vi "仁科设定参数对话框.vi"() -> ()   [LabVIEW 2016, in "环境动力监测库.lvlib" / "空调库.lvlib"]
panel:
  in  "帮助按钮":bool
  in  "时间 16":cluster{"小时":u16, "分钟":u16} {"分钟" format="%.0f分"; "小时" format="%.0f点"}
  in  "时间 15":cluster{"小时":u16, "分钟":u16} {"分钟" format="%.0f分"; "小时" format="%.0f点"}
  in  "时间 14":cluster{"小时":u16, "分钟":u16} {"分钟" format="%.0f分"; "小时" format="%.0f点"}
  in  "时间 13":cluster{"小时":u16, "分钟":u16} {"分钟" format="%.0f分"; "小时" format="%.0f点"}
  in  "时间 12":cluster{"小时":u16, "分钟":u16} {"分钟" format="%.0f分"; "小时" format="%.0f点"}
  in  "时间 11":cluster{"小时":u16, "分钟":u16} {"分钟" format="%.0f分"; "小时" format="%.0f点"}
  in  "时间 10":cluster{"小时":u16, "分钟":u16} {"分钟" format="%.0f分"; "小时" format="%.0f点"}
  in  "时间 9":cluster{"小时":u16, "分钟":u16} {"分钟" format="%.0f分"; "小时" format="%.0f点"}
  in  "时间 8":cluster{"小时":u16, "分钟":u16} {"分钟" format="%.0f分"; "小时" format="%.0f点"}
  in  "时间 7":cluster{"小时":u16, "分钟":u16} {"分钟" format="%.0f分"; "小时" format="%.0f点"}
  in  "时间 6":cluster{"小时":u16, "分钟":u16} {"分钟" format="%.0f分"; "小时" format="%.0f点"}
  in  "时间 5":cluster{"小时":u16, "分钟":u16} {"分钟" format="%.0f分"; "小时" format="%.0f点"}
  in  "时间 4":cluster{"小时":u16, "分钟":u16} {"分钟" format="%.0f分"; "小时" format="%.0f点"}
  in  "时间 3":cluster{"小时":u16, "分钟":u16} {"分钟" format="%.0f分"; "小时" format="%.0f点"}
  in  "时间 2":cluster{"小时":u16, "分钟":u16} {"分钟" format="%.0f分"; "小时" format="%.0f点"}
  in  "时间":cluster{"小时":u16, "分钟":u16} {"分钟" format="%.0f分"; "小时" format="%.0f点"}
  in  "通道2空调故障报警":bool
  in  "通道1空调故障报警":bool
  in  "低温报警":bool
  in  "超温报警":bool
  in  "空调电流门槛:":dbl
  in  "湿度偏差:":dbl
  in  "温度偏差:":dbl
  in  "自控温度回差:":dbl
  in  "自控温度下限:":dbl
  in  "温度报警下限:":dbl
  in  "自控温度上限:":dbl
  in  "温度报警上限:":dbl
  in  "切换时间(分钟):":dbl
  in  "双机切换":bool
  in  "控制模式:":enum16{"远程", "自动"}(ring)
  in  "来电自启":bool
  in  "写入控制参数":bool
  in  "读取运行参数":bool
  # "设定参数选择"
  # "通道运行时间段"
  # "时间段1"
  # "时间段2"
  # "时间段3"
  # "时间段4"
  # "通道1开始:"
  # "通道1结束:"
  # "通道2开始:"
  # "通道2结束:"
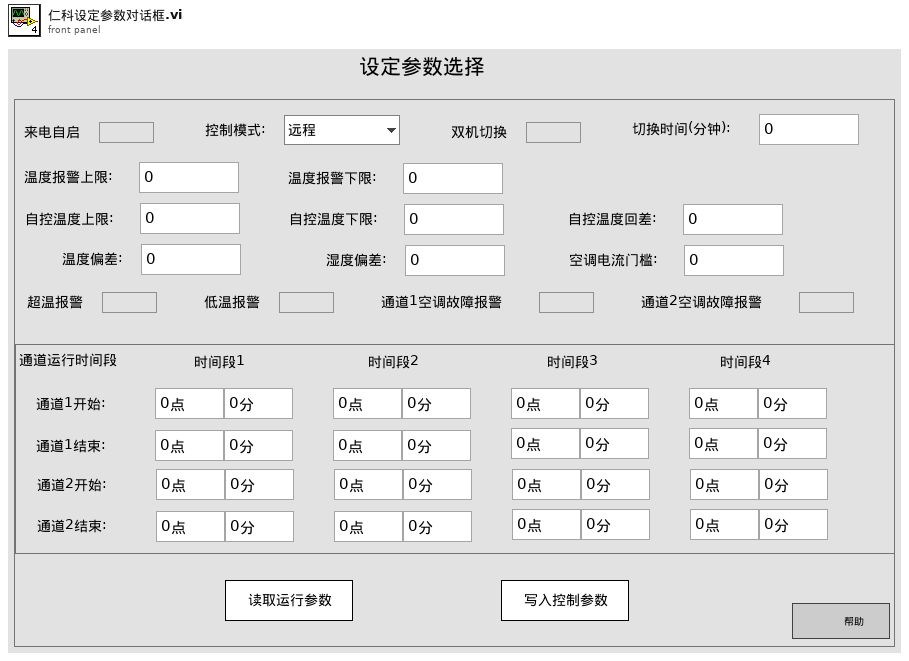
[diagram p1: front panel]
types:
  T1 = cluster{"来电自启":bool, "时间":cluster{"小时":u16, "分钟":u16}, "时间 2":cluster{"小时":u16, "分钟":u16}, "时间 3":cluster{"小时":u16, "分钟":u16}, "时间 4":cluster{"小时":u16, "分钟":u16}, "时间 5":cluster{"小时":u16, "分钟":u16}, "时间 6":cluster{"小时":u16, "分钟":u16}, "时间 7":cluster{"小时":u16, "分钟":u16}, "时间 8":cluster{"小时":u16, "分钟":u16}, "时间 9":cluster{"小时":u16, "分钟":u16}, "时间 10":cluster{"小时":u16, "分钟":u16}, "时间 11":cluster{"小时":u16, "分钟":u16}, "时间 12":cluster{"小时":u16, "分钟":u16}, "时间 13":cluster{"小时":u16, "分钟":u16}, "时间 14":cluster{"小时":u16, "分钟":u16}, "时间 15":cluster{"小时":u16, "分钟":u16}, "时间 16":cluster{"小时":u16, "分钟":u16}, "超温报警":bool, "低温报警":bool, "通道1空调故障报警":bool, "通道2空调故障报警":bool, "温度报警上限:":dbl, "温度报警下限:":dbl, "温度偏差:":dbl, "湿度偏差:":dbl, "自控温度上限:":dbl, "自控温度下限:":dbl, "自控温度回差:":dbl, "空调电流门槛:":dbl, "控制模式:":enum16{"远程", "自动"}, "双机切换":bool, "切换时间(分钟):":dbl}
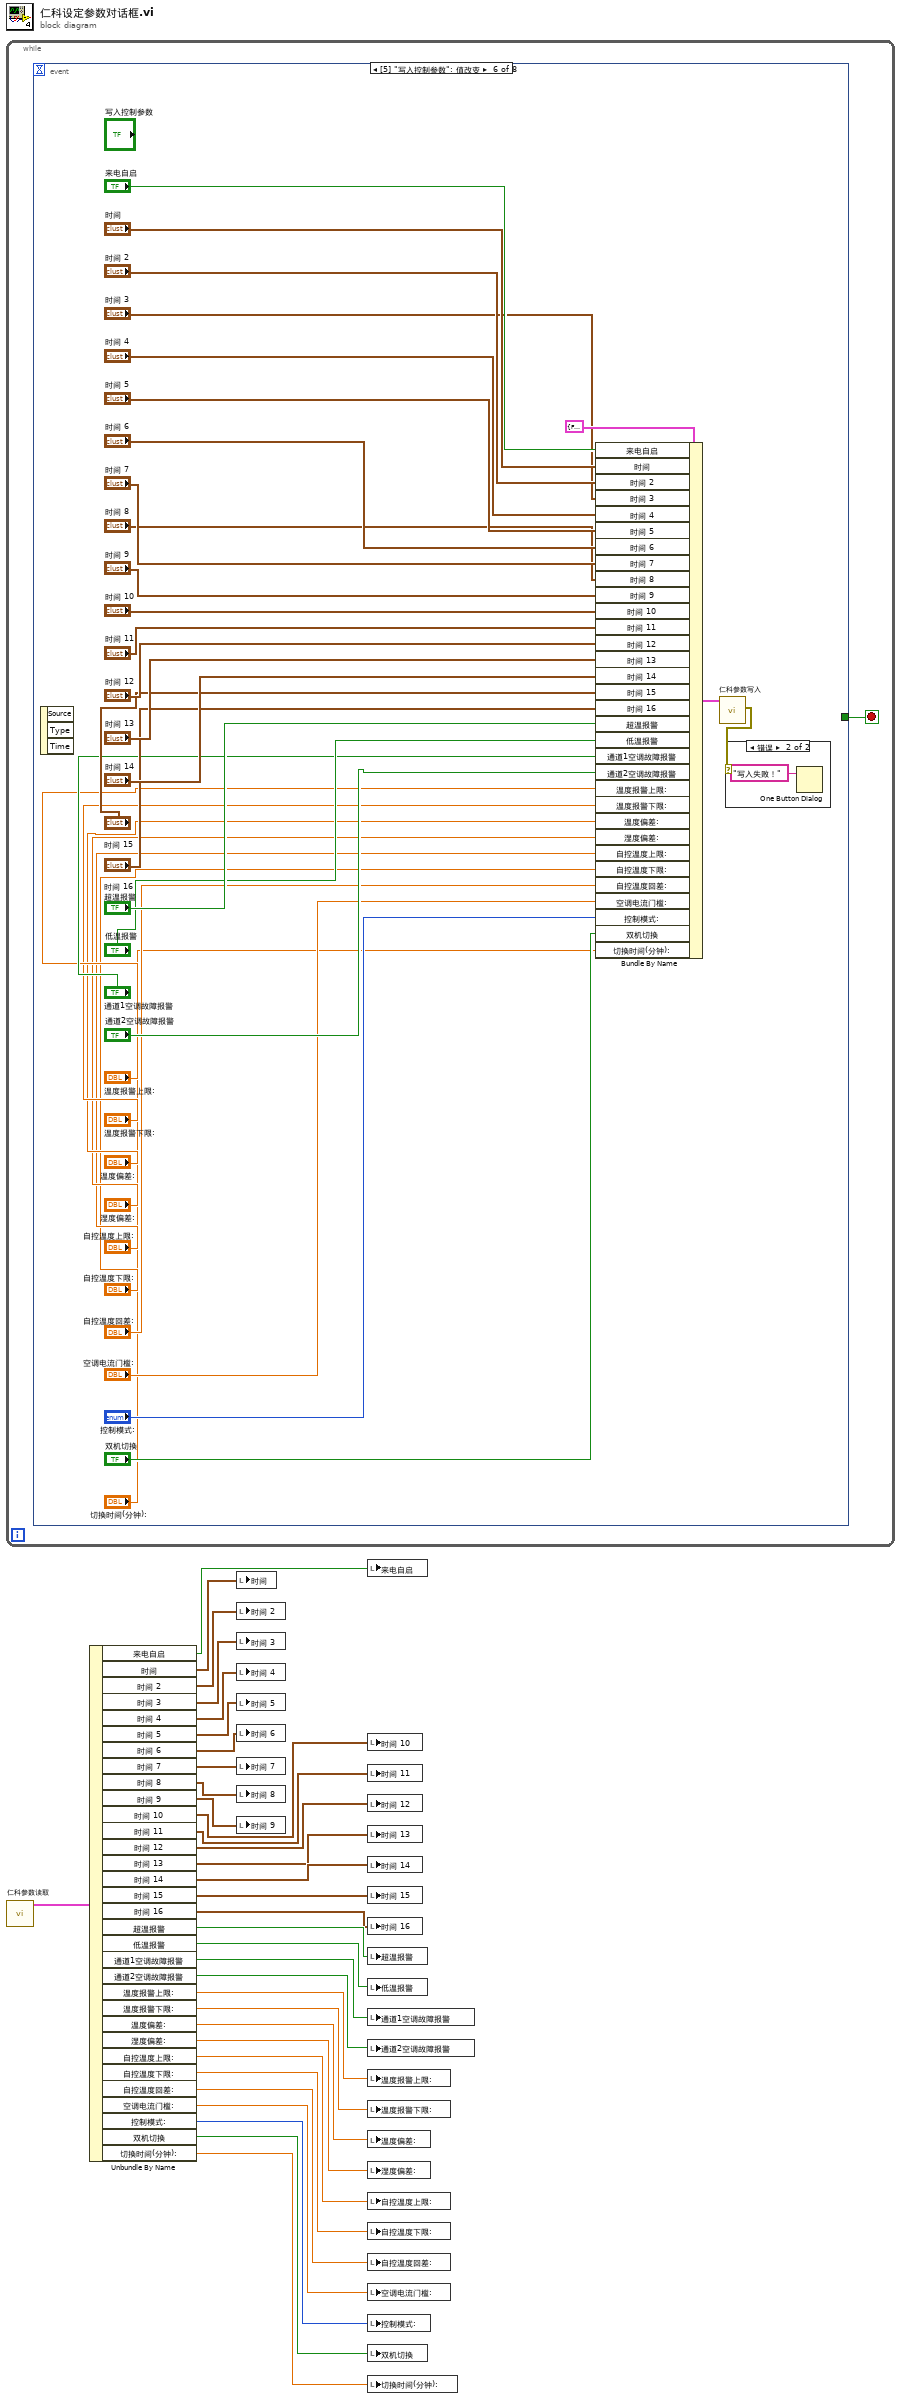
[diagram p0: block diagram]
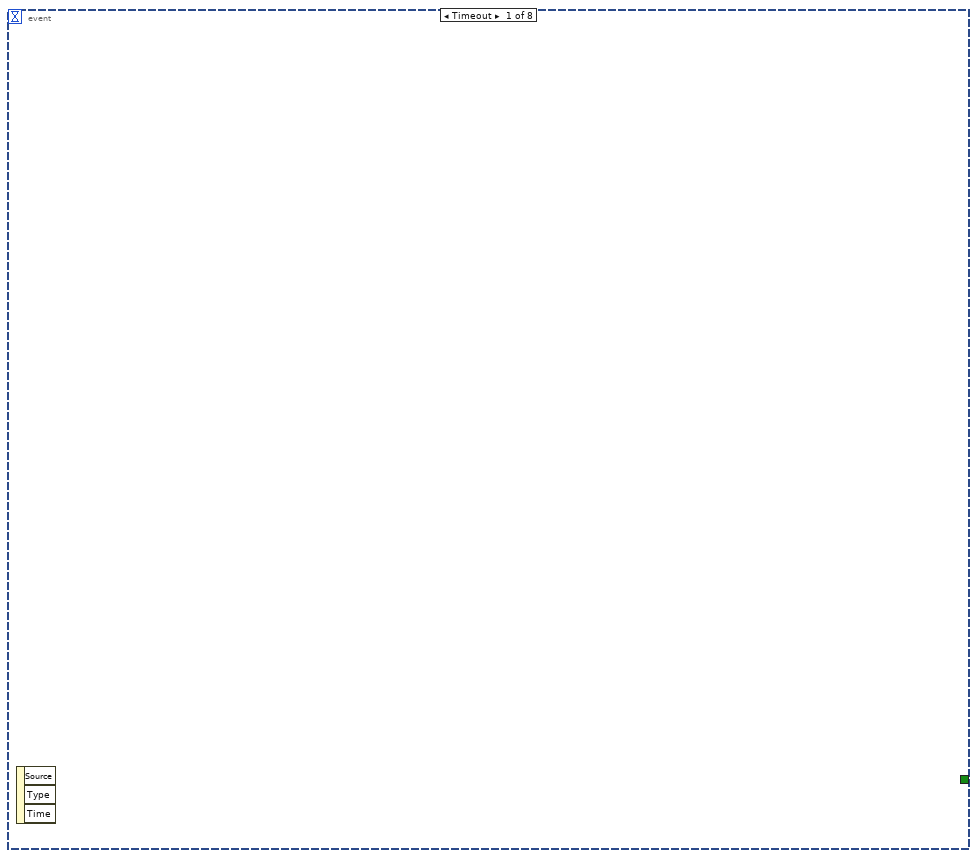
[diagram p2: hidden frame]
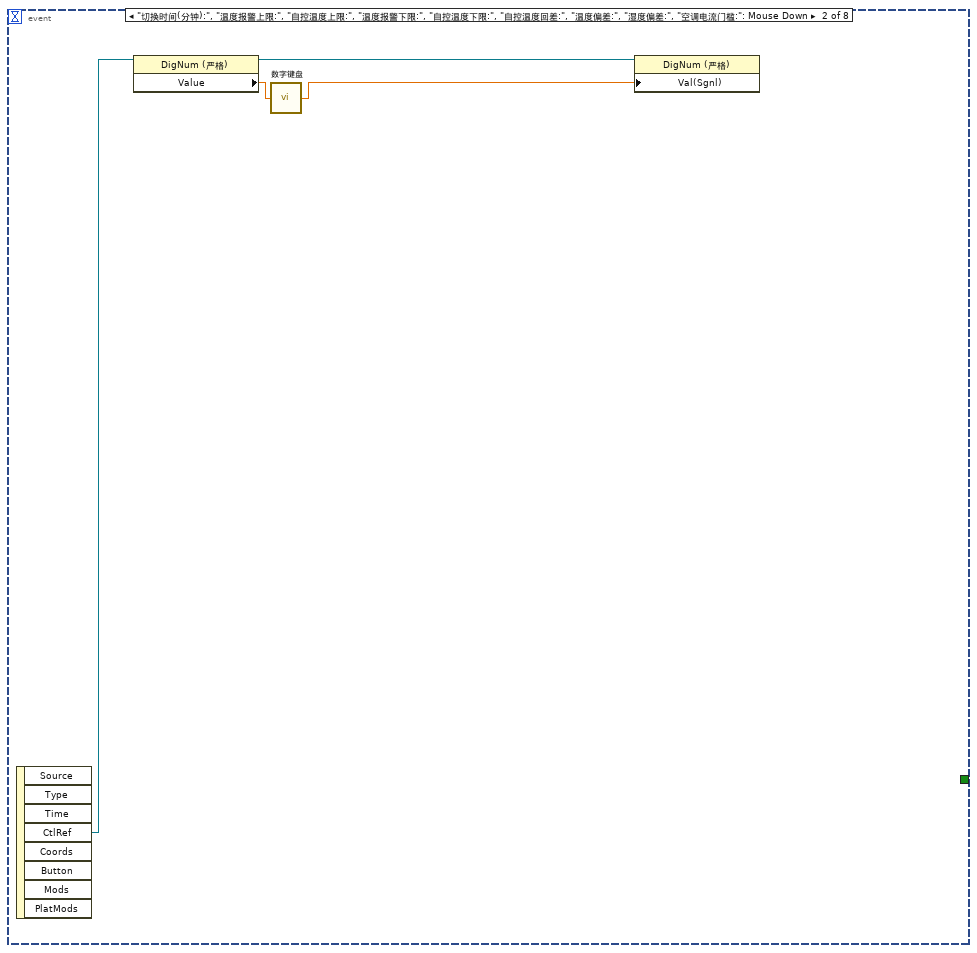
[diagram p3: hidden frame]
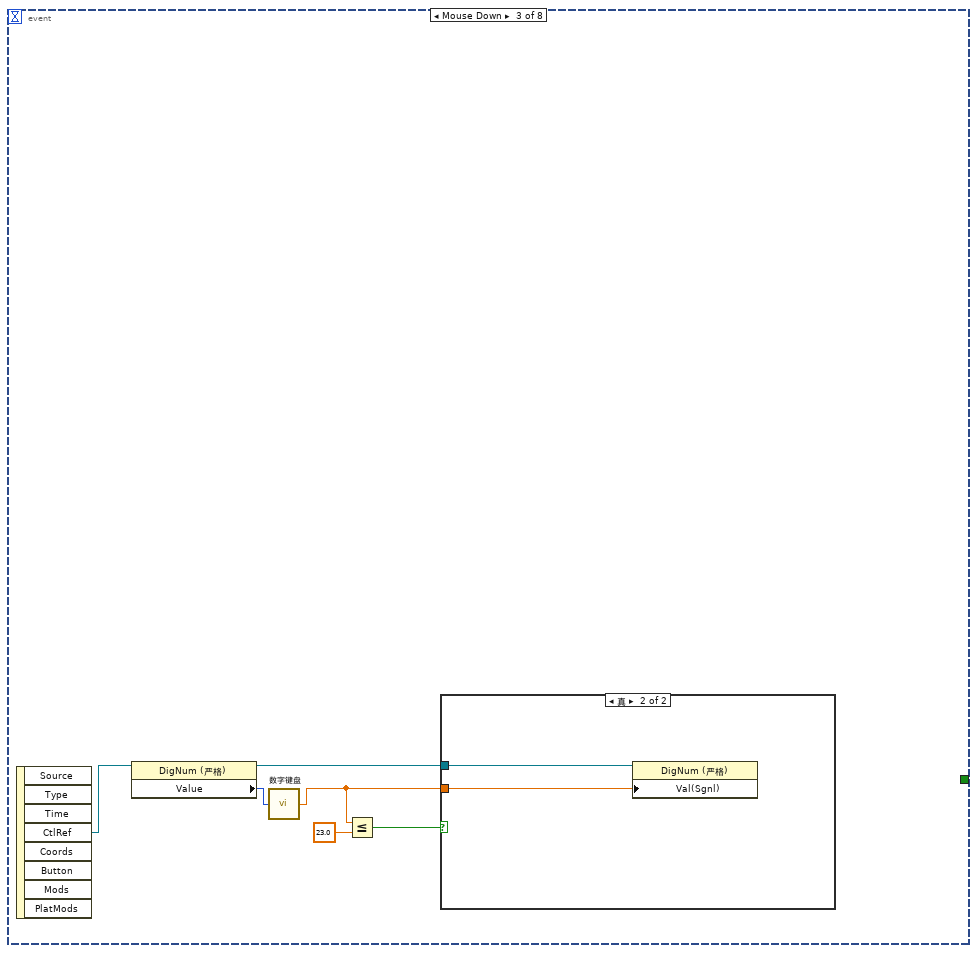
[diagram p4: hidden frame]
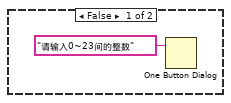
[diagram p5: hidden frame]
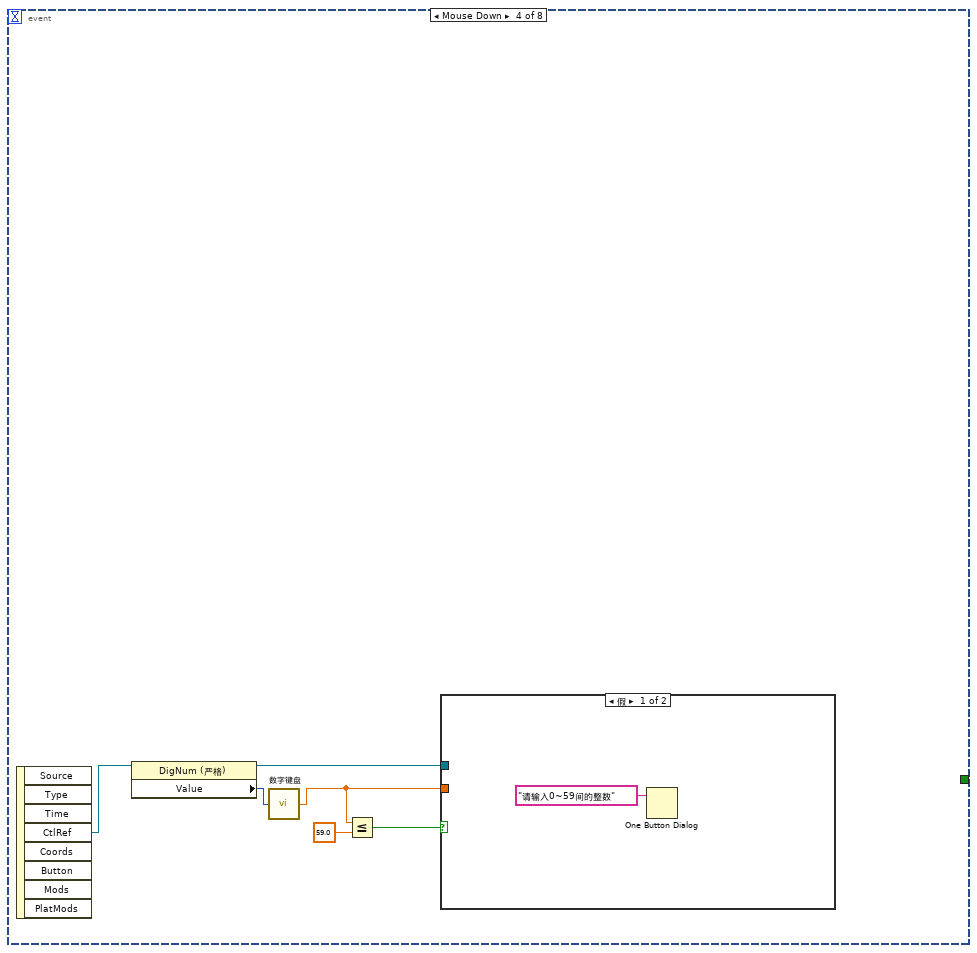
[diagram p6: hidden frame]
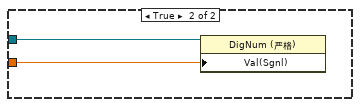
[diagram p7: hidden frame]
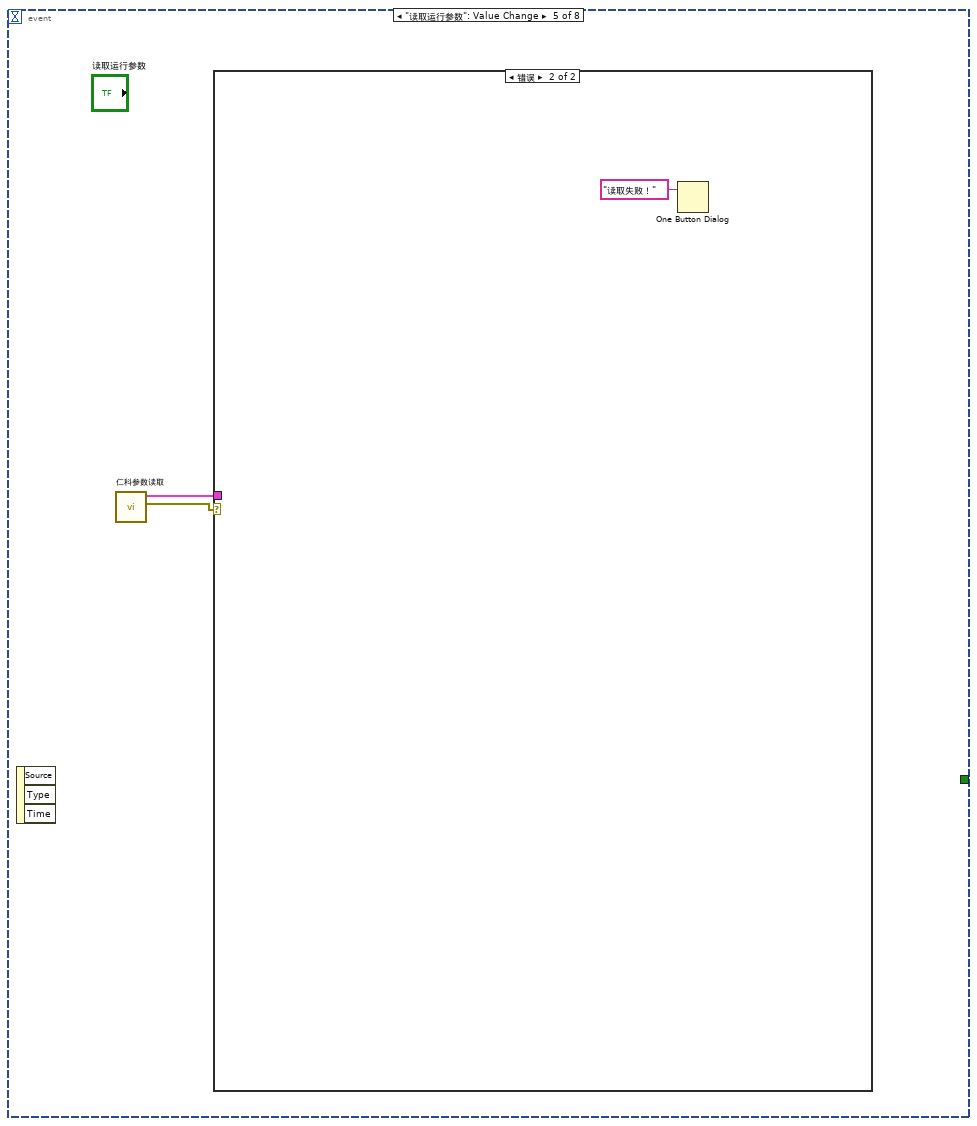
[diagram p8: hidden frame]
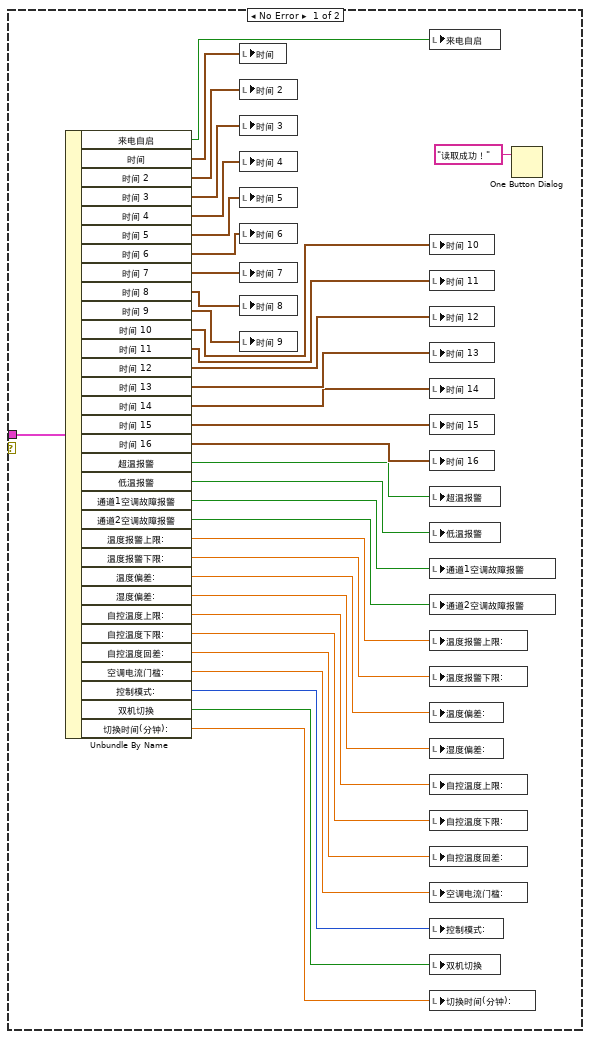
[diagram p9: hidden frame]
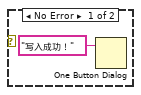
[diagram p10: hidden frame]
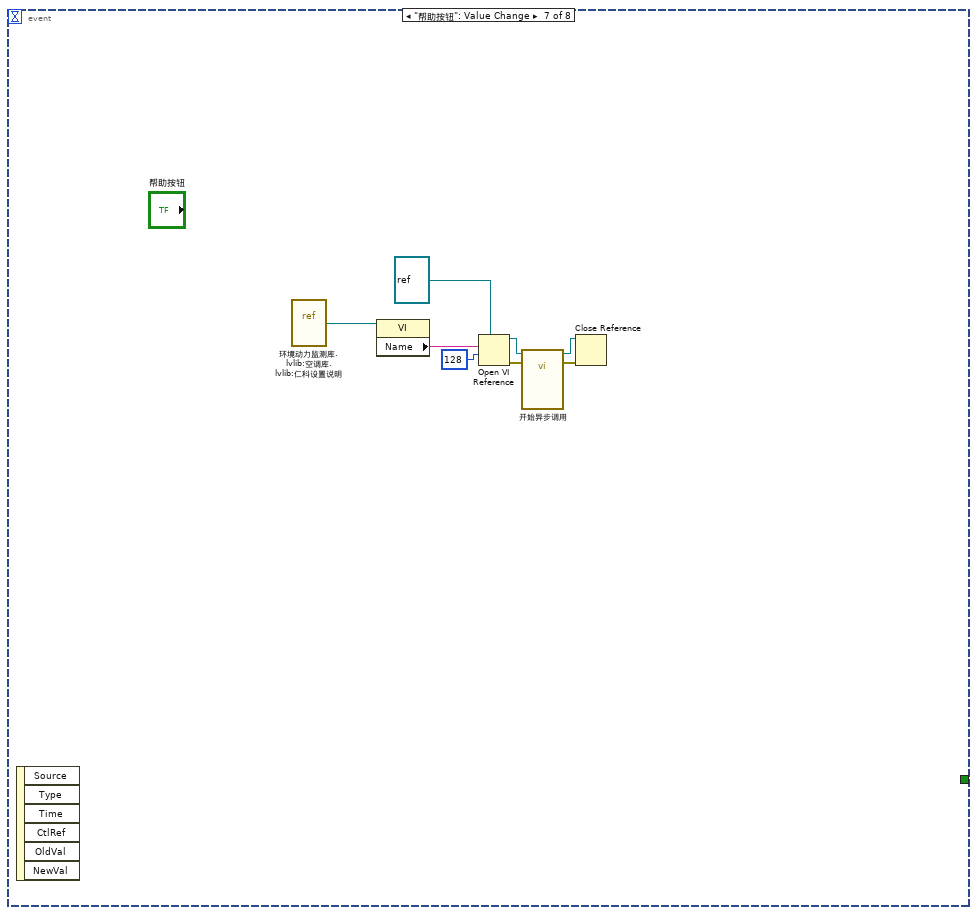
[diagram p11: hidden frame]
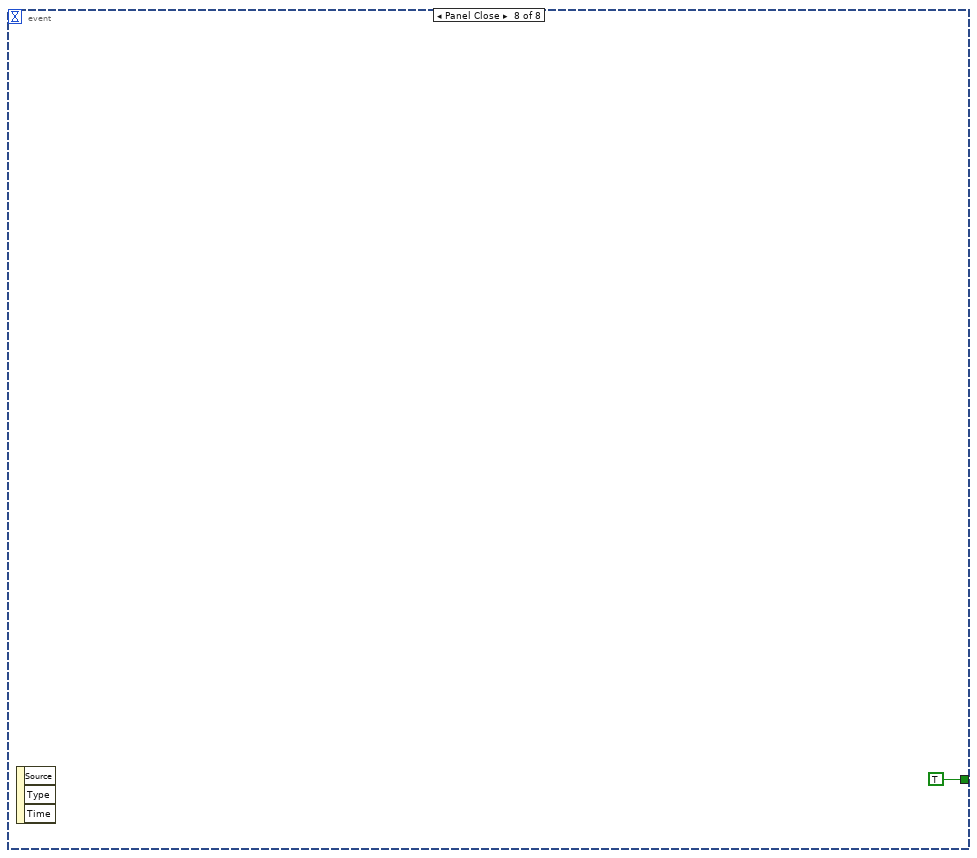
[diagram p12: hidden frame]
diagram:
  n1 = while {
    stop <- w34 stop-if-true
    n2 = event shown="[5] \"写入控制参数\": 值改变" {
      selector: _ -> [_ _ _ _ _ _ _ _]
      dyn-events: _ -> [_ _ _ _ _ _ _ _]
      timeout: _ -> [_ _ _ _ _ _ _ _]
      tunnel: [_ _ _ _ _ _ _ TRUE] -> w34
      event Timeout {
        n3 = event-data() -> ()  [unwired: 1 in, 3 out]
      }
      event "切换时间(分钟):", "温度报警上限:", "自控温度上限:", "温度报警下限:", "自控温度下限:", "自控温度回差:", "温度偏差:", "湿度偏差:", "空调电流门槛:": Mouse Down {
        n4 = event-data() -> ("CtlRef"=w35:refnum<vi>)  [unwired: 1 in, 7 out]
        n5 = property class="DigNum (严格)"(reference=w35) -> (reference out=w36:refnum<vi>, "Value"=w38:dbl)  [unwired: 1 in, 1 out]
        n6 = call "数字键盘.vi"("OldNumber"=w38) -> ("NewNumber"=w37:sgl)
        n7 = property class="DigNum (严格)"(reference=w36, "Val(Sgnl)"=w37) -> ()  [unwired: 1 in, 2 out]
      }
      event "时间.小时", "时间 2.小时", "时间 3.小时", "时间 4.小时", "时间 5.小时", "时间 6.小时", "时间 7.小时", "时间 8.小时", "时间 9.小时", "时间 10.小时", "时间 11.小时", "时间 12.小时", "时间 13.小时", "时间 14.小时", "时间 15.小时", "时间 16.小时": Mouse Down {
        n8 = event-data() -> ("CtlRef"=w42:refnum<vi>)  [unwired: 1 in, 7 out]
        n9 = property class="DigNum (严格)"(reference=w42) -> (reference out=w43:refnum<vi>, "Value"=w44:u16)  [unwired: 1 in, 1 out]
        n10 = call "数字键盘.vi"("OldNumber"=w44) -> ("NewNumber"=w41:sgl)
        n11 = Less Or Equal?(x=w41, y=sgl 23.0) -> (x <= y?=w39:bool)
        n12 = case shown="真" w39 {
          tunnel: w41 -> [_ w47]
          tunnel: w43 -> [_ w46]
          frame False {
            n13 = One Button Dialog(message="请输入0~23间的整数" ("消息")) -> ()  [unwired: 1 in, 1 out]
          }
          frame True {
            n14 = property class="DigNum (严格)"(reference=w46, "Val(Sgnl)"=w47) -> ()  [unwired: 1 in, 2 out]
          }
        }
      }
      event "时间.分钟", "时间 2.分钟", "时间 3.分钟", "时间 4.分钟", "时间 5.分钟", "时间 6.分钟", "时间 7.分钟", "时间 8.分钟", "时间 9.分钟", "时间 10.分钟", "时间 11.分钟", "时间 12.分钟", "时间 13.分钟", "时间 14.分钟", "时间 15.分钟", "时间 16.分钟": Mouse Down {
        n15 = event-data() -> ("CtlRef"=w51:refnum<vi>)  [unwired: 1 in, 7 out]
        n16 = property class="DigNum (严格)"(reference=w51) -> (reference out=w52:refnum<vi>, "Value"=w53:u16)  [unwired: 1 in, 1 out]
        n17 = call "数字键盘.vi"("OldNumber"=w53) -> ("NewNumber"=w50:sgl)
        n18 = Less Or Equal?(x=w50, y=sgl 59.0) -> (x <= y?=w48:bool)
        n19 = case shown="假" w48 {
          tunnel: w50 -> [_ w56]
          tunnel: w52 -> [_ w55]
          frame False {
            n20 = One Button Dialog(message="请输入0~59间的整数" ("消息")) -> ()  [unwired: 1 in, 1 out]
          }
          frame True {
            n21 = property class="DigNum (严格)"(reference=w55, "Val(Sgnl)"=w56) -> ()  [unwired: 1 in, 2 out]
          }
        }
      }
      event "读取运行参数": Value Change {
        n22 = event-data() -> ()  [unwired: 1 in, 3 out]
        n23 = call "仁科参数读取.vi"() -> ("error out"=w57:errorcluster, "簇"=w58:T1)  [unwired: 10 in]
        n24 = case shown="错误" w57 {
          tunnel: w58 -> [w92 _]
          frame No Error {
            n25 = Unbundle By Name(w92) -> ("来电自启"=w91:bool, "时间"=w90:cluster{"小时":u16, "分钟":u16}, "时间 2"=w89:cluster{"小时":u16, "分钟":u16}, "时间 3"=w88:cluster{"小时":u16, "分钟":u16}, "时间 4"=w87:cluster{"小时":u16, "分钟":u16}, "时间 5"=w86:cluster{"小时":u16, "分钟":u16}, "时间 6"=w85:cluster{"小时":u16, "分钟":u16}, "时间 7"=w84:cluster{"小时":u16, "分钟":u16}, "时间 8"=w83:cluster{"小时":u16, "分钟":u16}, "时间 9"=w82:cluster{"小时":u16, "分钟":u16}, "时间 10"=w81:cluster{"小时":u16, "分钟":u16}, "时间 11"=w80:cluster{"小时":u16, "分钟":u16}, "时间 12"=w79:cluster{"小时":u16, "分钟":u16}, "时间 13"=w78:cluster{"小时":u16, "分钟":u16}, "时间 14"=w77:cluster{"小时":u16, "分钟":u16}, "时间 15"=w76:cluster{"小时":u16, "分钟":u16}, "时间 16"=w75:cluster{"小时":u16, "分钟":u16}, "超温报警"=w74:bool, "低温报警"=w73:bool, "通道1空调故障报警"=w72:bool, "通道2空调故障报警"=w71:bool, "温度报警上限:"=w70:dbl, "温度报警下限:"=w69:dbl, "温度偏差:"=w68:dbl, "湿度偏差:"=w67:dbl, "自控温度上限:"=w66:dbl, "自控温度下限:"=w65:dbl, "自控温度回差:"=w64:dbl, "空调电流门槛:"=w63:dbl, "控制模式:"=w62:enum16{"远程", "自动"}, "双机切换"=w61:bool, "切换时间(分钟):"=w60:dbl)
            n26 = local write "时间"(w90) -> ()
            n27 = local write "时间 2"(w89) -> ()
            n28 = local write "时间 3"(w88) -> ()
            n29 = local write "时间 4"(w87) -> ()
            n30 = local write "时间 5"(w86) -> ()
            n31 = local write "时间 6"(w85) -> ()
            n32 = local write "时间 7"(w84) -> ()
            n33 = local write "时间 8"(w83) -> ()
            n34 = local write "时间 9"(w82) -> ()
            n35 = local write "来电自启"(w91) -> ()
            n36 = local write "时间 10"(w81) -> ()
            n37 = local write "时间 11"(w80) -> ()
            n38 = local write "时间 12"(w79) -> ()
            n39 = local write "时间 13"(w78) -> ()
            n40 = local write "时间 14"(w77) -> ()
            n41 = local write "时间 15"(w76) -> ()
            n42 = local write "时间 16"(w75) -> ()
            n43 = local write "超温报警"(w74) -> ()
            n44 = local write "低温报警"(w73) -> ()
            n45 = local write "通道1空调故障报警"(w72) -> ()
            n46 = local write "通道2空调故障报警"(w71) -> ()
            n47 = local write "温度报警上限:"(w70) -> ()
            n48 = local write "温度报警下限:"(w69) -> ()
            n49 = local write "温度偏差:"(w68) -> ()
            n50 = local write "湿度偏差:"(w67) -> ()
            n51 = local write "自控温度上限:"(w66) -> ()
            n52 = local write "自控温度下限:"(w65) -> ()
            n53 = local write "自控温度回差:"(w64) -> ()
            n54 = local write "空调电流门槛:"(w63) -> ()
            n55 = local write "控制模式:"(w62) -> ()
            n56 = local write "双机切换"(w61) -> ()
            n57 = local write "切换时间(分钟):"(w60) -> ()
            n58 = One Button Dialog(message="读取成功！" ("消息")) -> ()  [unwired: 1 in, 1 out]
          }
          frame Error {
            n59 = One Button Dialog(message="读取失败！" ("消息")) -> ()  [unwired: 1 in, 1 out]
          }
        }
      }
      event "写入控制参数": Value Change {
        n60 = event-data() -> ()  [unwired: 1 in, 3 out]
        n61 = Bundle By Name(cluster=T1 {"来电自启"=FALSE, "时间"={"小时"=0, "分钟"=0}, "时间 2"={"小时"=0, "分钟"=0}, "时间 3"={"小时"=0, "分钟"=0}, "时间 4"={"小时"=0, "分钟"=0}, "时间 5"={"小时"=0, "分钟"=0}, "时间 6"={"小时"=0, "分钟"=0}, "时间 7"={"小时"=0, "分钟"=0}, "时间 8"={"小时"=0, "分钟"=0}, "时间 9"={"小时"=0, "分钟"=0}, "时间 10"={"小时"=0, "分钟"=0}, "时间 11"={"小时"=0, "分钟"=0}, "时间 12"={"小时"=0, "分钟"=0}, "时间 13"={"小时"=0, "分钟"=0}, "时间 14"={"小时"=0, "分钟"=0}, "时间 15"={"小时"=0, "分钟"=0}, "时间 16"={"小时"=0, "分钟"=0}, "超温报警"=FALSE, "低温报警"=FALSE, "通道1空调故障报警"=FALSE, "通道2空调故障报警"=FALSE, "温度报警上限:"=0.0, "温度报警下限:"=0.0, "温度偏差:"=0.0, "湿度偏差:"=0.0, "自控温度上限:"=0.0, "自控温度下限:"=0.0, "自控温度回差:"=0.0, "空调电流门槛:"=0.0, "控制模式:"=enum."远程", "双机切换"=FALSE, "切换时间(分钟):"=0.0} ("簇"), "来电自启"="来电自启", "时间"="时间", "时间 2"="时间 2", "时间 3"="时间 3", "时间 4"="时间 4", "时间 5"="时间 5", "时间 6"="时间 6", "时间 7"="时间 7", "时间 8"="时间 8", "时间 9"="时间 9", "时间 10"="时间 10", "时间 11"="时间 11", "时间 12"="时间 12", "时间 13"="时间 13", "时间 14"="时间 14", "时间 15"="时间 15", "时间 16"="时间 16", "超温报警"="超温报警", "低温报警"="低温报警", "通道1空调故障报警"="通道1空调故障报警", "通道2空调故障报警"="通道2空调故障报警", "温度报警上限:"="温度报警上限:", "温度报警下限:"="温度报警下限:", "温度偏差:"="温度偏差:", "湿度偏差:"="湿度偏差:", "自控温度上限:"="自控温度上限:", "自控温度下限:"="自控温度下限:", "自控温度回差:"="自控温度回差:", "空调电流门槛:"="空调电流门槛:", "控制模式:"="控制模式:", "双机切换"="双机切换", "切换时间(分钟):"="切换时间(分钟):") -> (w127:T1)
        n62 = call "仁科参数写入.vi"("簇"=w127) -> ("error out"=w94:errorcluster)  [unwired: 10 in]
        n63 = case shown="错误" w94 {
          frame No Error {
            n64 = One Button Dialog(message="写入成功！" ("消息")) -> ()  [unwired: 1 in, 1 out]
          }
          frame Error {
            n65 = One Button Dialog(message="写入失败！" ("消息")) -> ()  [unwired: 1 in, 1 out]
          }
        }
      }
      event "帮助按钮": Value Change {
        n66 = event-data() -> ()  [unwired: 1 in, 6 out]
        n67 = vi-ref "环境动力监测库.lvlib:空调库.lvlib:仁科设置说明.vi"() -> (w131:refnum<vi>)
        n68 = property class="VI"(reference=w131) -> ("Name"=w132:string)  [unwired: 1 in, 2 out]
        n69 = Open VI Reference(type specifier VI Refnum (for type only)=refnum<vi> refnum, vi path=w132, options=128 ("选项")) -> (vi reference=w134:refnum<vi>, error out=w136:errorcluster)  [unwired: 3 in]
        n70 = call-by-ref "开始异步调用"(reference=w134, error in=w136) -> (reference out=w138:refnum<vi>, error out=w137:errorcluster)  [unwired: 11 in, 1 out]
        n71 = Close Reference(reference=w138, error in (no error)=w137) -> ()  [unwired: 1 out]
      }
      event Panel Close {
        n72 = event-data() -> ()  [unwired: 1 in, 3 out]
      }
    }
  }
  n73 = call "仁科参数读取.vi"() -> ("簇"=w1:T1)  [unwired: 10 in, 1 out]
  n74 = Unbundle By Name(w1) -> ("来电自启"=w2:bool, "时间"=w3:cluster{"小时":u16, "分钟":u16}, "时间 2"=w4:cluster{"小时":u16, "分钟":u16}, "时间 3"=w5:cluster{"小时":u16, "分钟":u16}, "时间 4"=w6:cluster{"小时":u16, "分钟":u16}, "时间 5"=w7:cluster{"小时":u16, "分钟":u16}, "时间 6"=w8:cluster{"小时":u16, "分钟":u16}, "时间 7"=w9:cluster{"小时":u16, "分钟":u16}, "时间 8"=w10:cluster{"小时":u16, "分钟":u16}, "时间 9"=w11:cluster{"小时":u16, "分钟":u16}, "时间 10"=w12:cluster{"小时":u16, "分钟":u16}, "时间 11"=w13:cluster{"小时":u16, "分钟":u16}, "时间 12"=w14:cluster{"小时":u16, "分钟":u16}, "时间 13"=w15:cluster{"小时":u16, "分钟":u16}, "时间 14"=w16:cluster{"小时":u16, "分钟":u16}, "时间 15"=w17:cluster{"小时":u16, "分钟":u16}, "时间 16"=w18:cluster{"小时":u16, "分钟":u16}, "超温报警"=w19:bool, "低温报警"=w20:bool, "通道1空调故障报警"=w21:bool, "通道2空调故障报警"=w22:bool, "温度报警上限:"=w23:dbl, "温度报警下限:"=w24:dbl, "温度偏差:"=w25:dbl, "湿度偏差:"=w26:dbl, "自控温度上限:"=w27:dbl, "自控温度下限:"=w28:dbl, "自控温度回差:"=w29:dbl, "空调电流门槛:"=w30:dbl, "控制模式:"=w31:enum16{"远程", "自动"}, "双机切换"=w32:bool, "切换时间(分钟):"=w33:dbl)
  n75 = local write "时间"(w3) -> ()
  n76 = local write "时间 2"(w4) -> ()
  n77 = local write "时间 3"(w5) -> ()
  n78 = local write "时间 4"(w6) -> ()
  n79 = local write "时间 5"(w7) -> ()
  n80 = local write "时间 6"(w8) -> ()
  n81 = local write "时间 7"(w9) -> ()
  n82 = local write "时间 8"(w10) -> ()
  n83 = local write "时间 9"(w11) -> ()
  n84 = local write "来电自启"(w2) -> ()
  n85 = local write "时间 10"(w12) -> ()
  n86 = local write "时间 11"(w13) -> ()
  n87 = local write "时间 12"(w14) -> ()
  n88 = local write "时间 13"(w15) -> ()
  n89 = local write "时间 14"(w16) -> ()
  n90 = local write "时间 15"(w17) -> ()
  n91 = local write "时间 16"(w18) -> ()
  n92 = local write "超温报警"(w19) -> ()
  n93 = local write "低温报警"(w20) -> ()
  n94 = local write "通道1空调故障报警"(w21) -> ()
  n95 = local write "通道2空调故障报警"(w22) -> ()
  n96 = local write "温度报警上限:"(w23) -> ()
  n97 = local write "温度报警下限:"(w24) -> ()
  n98 = local write "温度偏差:"(w25) -> ()
  n99 = local write "湿度偏差:"(w26) -> ()
  n100 = local write "自控温度上限:"(w27) -> ()
  n101 = local write "自控温度下限:"(w28) -> ()
  n102 = local write "自控温度回差:"(w29) -> ()
  n103 = local write "空调电流门槛:"(w30) -> ()
  n104 = local write "控制模式:"(w31) -> ()
  n105 = local write "双机切换"(w32) -> ()
  n106 = local write "切换时间(分钟):"(w33) -> ()
